vi "Delacor_lib_QMH_Error Handler - Helper Loop.vi"(6 "HelperName":string, 7 "Error Message Name (\"Error\")":string="Error", 8 "error in":errorcluster, 10 "Ignore Errors (Runtime)":i32[](array[numeric]), 11 "Message Queue in":refnum<class "RQMHMessageQueue.lvclass">) -> (0 "dup error in":errorcluster, 3 "Message Queue out":refnum<class "RQMHMessageQueue.lvclass">)   [LabVIEW 2024, in "RQMHMessageQueue.lvclass"]
doc: "Process an error that occurred in a Helper Loop, either by ignoring it, or generating an \"Error\" message.\n____\nDQMH Framework: Palette 7.1.0.1503\nCopyright (c) 2025, DQMH Consortium"
uses:
  RQMHMessageQueue.lvclass
  RQMHMessageQueue.lvclass/RQMHMessageQueue.ctl
  Delacor_lib_QMH_Set Error Debug.vi
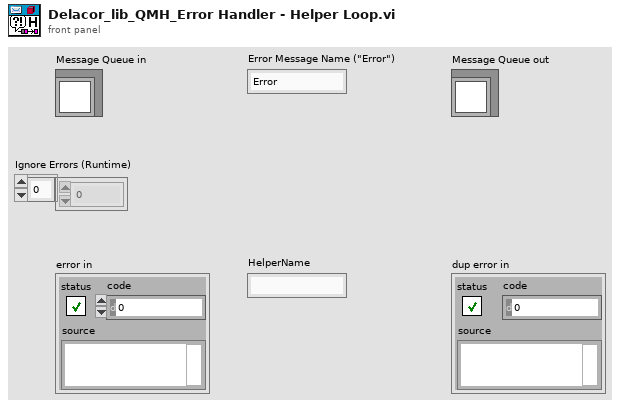
[diagram p1: front panel]
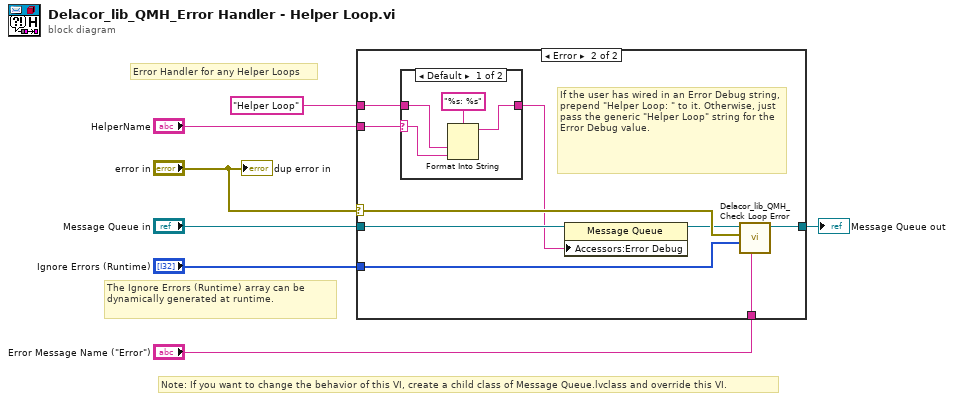
[diagram p0: block diagram]
diagram:
  # "Note: If you want to change the behavior of this VI, create a child class of Message Queue.lvclass and override this VI."
  # "The Ignore Errors (Runtime) array can be dynamically generated at runtime."
  # "Error Handler for any Helper Loops"
  n1 = case shown="Error" "error in" {
    selector: "error in" -> [_ w17]
    tunnel: "Message Queue in" -> [w8 w16]
    tunnel: "Ignore Errors (Runtime)" -> [_ w15]
    tunnel: [w8 w14] -> w4
    tunnel: "Error Message Name (\"Error\")" -> [_ w13]
    tunnel: "HelperName" -> [_ w11]
    tunnel: "Helper Loop" -> [_ w10]
    frame No Error {
    }
    frame Error {
      # "If the user has wired in an Error Debug string, prepend \"Helper Loop: \" to it. Otherwise, just pass the generic \"Helper Loop\" string for the Error Debug value."
      n2 = case shown="Default" w11 {
        selector: w11 -> [w19 _]
        tunnel: w10 -> [w20 w22]
        tunnel: [w18 w22] -> w9
        frame Default {
          n3 = Format Into String(format string="%s: %s", w20, w19) -> (resulting string=w18:string)  [unwired: 2 in, 1 out]
        }
        frame "" {
        }
      }
      n4 = property class="Message Queue"(reference=w16, "Accessors:Error Debug"=w9) -> (reference out=w12:refnum<class "RQMHMessageQueue.lvclass">)  [unwired: 1 in, 1 out]
      n5 = call-dynamic "Delacor_lib_QMH_Check Loop Error.vi"("Error Message Name (\"Error\")"=w13, "Ignore Errors"=w15, "error to process"=w17, "Message Queue in"=w12) -> ("Message Queue out"=w14:refnum<class "RQMHMessageQueue.lvclass">)  [unwired: 6 in, 1 out]
    }
  }
  "Message Queue out" <- w4
  "dup error in" <- "error in"
